vi "Motor_Plus_Impedance_controller_thursday.vi"() -> ()   [LabVIEW 2016]
uses:
  <vilib>/Platform/TimedLoop/XDataNode/timing_clust.ctl
  <vilib>/Platform/TimedLoop/XDataNode/nitl_modes.ctl
  <vilib>/Platform/TimedLoop/XDataNode/wakeup.ctl
  <vilib>/Platform/TimedLoop/XDataNode/loadnilvce.vi
  <vilib>/Motion/Express/_s/nimc.ax.power.power.axis.vi
  <vilib>/Motion/Express/_s/nimc.fb.read.readExecutionData.axis.vi
  <vilib>/Motion/Express/_s/nimc.fb.straightLineMove.startStraightLineMove.axis.modeVelocity.0.vi
  <vilib>/Motion/Express/_s/nimc.fb.stopMove.stop.axis.modeDecelerate.vi
  <vilib>/Motion/Express/_s/nimc.fb.resetPosition.resetPosition.axis.vi
  <vilib>/Motion/Express/_s/nimc.ex.power.power.axis.vi
  <vilib>/platform/TimedLoop/XDataNode/XDataNode.xnode
  <vilib>/Motion/BlockNode/FB.NIMotion.xnode
  <vilib>/Platform/TimedLoop/XDataNode/XDNodeRunTimeDep.lvlib
panel:
  in  "Exo Force 2":dbl=0.25 format="%#_13g"
  in  "Speed 2":dbl=0.25 format="%#_13g"
  in  "Position 2":dbl=0.25 format="%#_13g"
  in  "Exo Force":dbl=0.25 format="%#_13g"
  out "Adjusted Motor Velocity":dbl format="%.3f"
  out "Adjusted Velocity":dbl(knob) scale=0.0..3.0
  in  "Reset Position":bool
  in  "Position":dbl=0.25 format="%#_13g"
  in  "Speed":dbl=0.25 format="%#_13g"
  out "Torque":dbl(knob) scale=-5.0..5.0
  out "Position":dbl(knob) scale=0.0..1.0
  out "Velocity":dbl(knob) scale=0.0..5.0
  out "Load Cell":dbl(knob) scale=0.0..10.0
  in  "Move to Position?":bool
  out "Load cell, V":dbl format="%.3f"
  out "motor torque, Nm":dbl format="%.3f"
  out "motor velocity, rev/s":dbl format="%.3f"
  out "motor position, rev":dbl format="%.3f"
  in  "STOP VI":bool
  in  "Enable Axis \nControl":bool
  in  "Enable Motor \nDrive":bool
  in  "EMERGENCY MOTOR STOP":bool
  # "Raw Data from System"
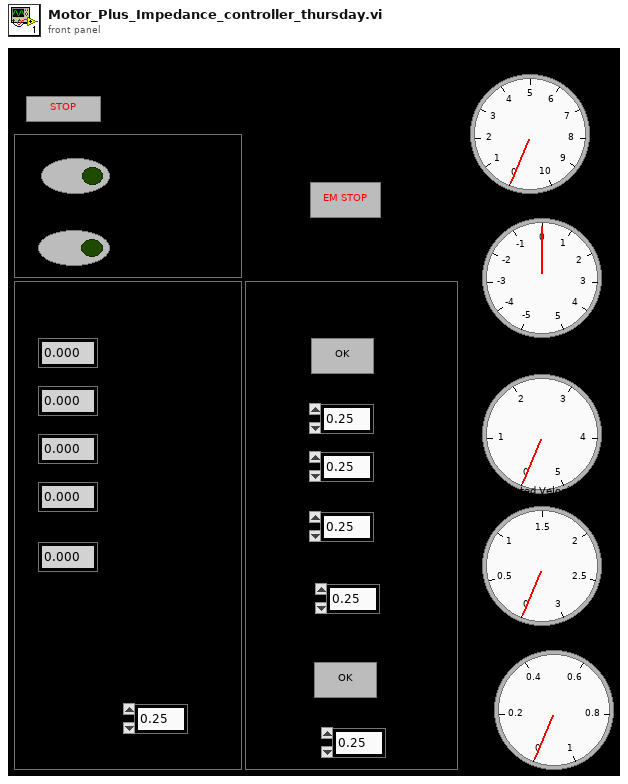
[diagram p1: front panel]
types:
  T1 = typedef "XDNodeRunTimeDep.lvlib/timing_clust.ctl" = cluster{"Expected End [f-1]":u64, "Actual End [f-1]":u64, "Finished Late? [f-1]":bool, "Expected End [i-1]":u64, "Actual End [i-1]":u64, "Finished Late? [i-1]":bool, "Expected Start [i]":u64, "Actual Start [i]":u64, "Expected Start [f]":u64, "Actual Start [f]":u64, "Source Name":string, "Structure Name":string, "Period":i64, "Deadline":i64, "Offset":i64, "Start":i64, "Priority":i32, "Timeout":i32, "Mode":T2, "Wakeup Reason":T3, "Error":errorcluster, "Source Type":string, "Secondary Source Type":string, "Global End Time":u64, "Global Start Time":u64, "Frame Duration":u64, "Iteration Duration":u64, "Assigned CPU":i32, "I/O Scan Engine Mode":u32}
  T2 = typedef "XDNodeRunTimeDep.lvlib/nitl_modes.ctl" = enum32{"No Change", "Process missed periods, maintain original phase", "Discard missed periods, maintain original phase", "Process missed periods, ignore original phase", "Discard missed periods, ignore original phase"}
  T3 = typedef "XDNodeRunTimeDep.lvlib/wakeup.ctl" = enum32{"Normal", "Aborted", "Asynchronous wakeup", "Timing source error", "Timed loop error", "Timeout"}
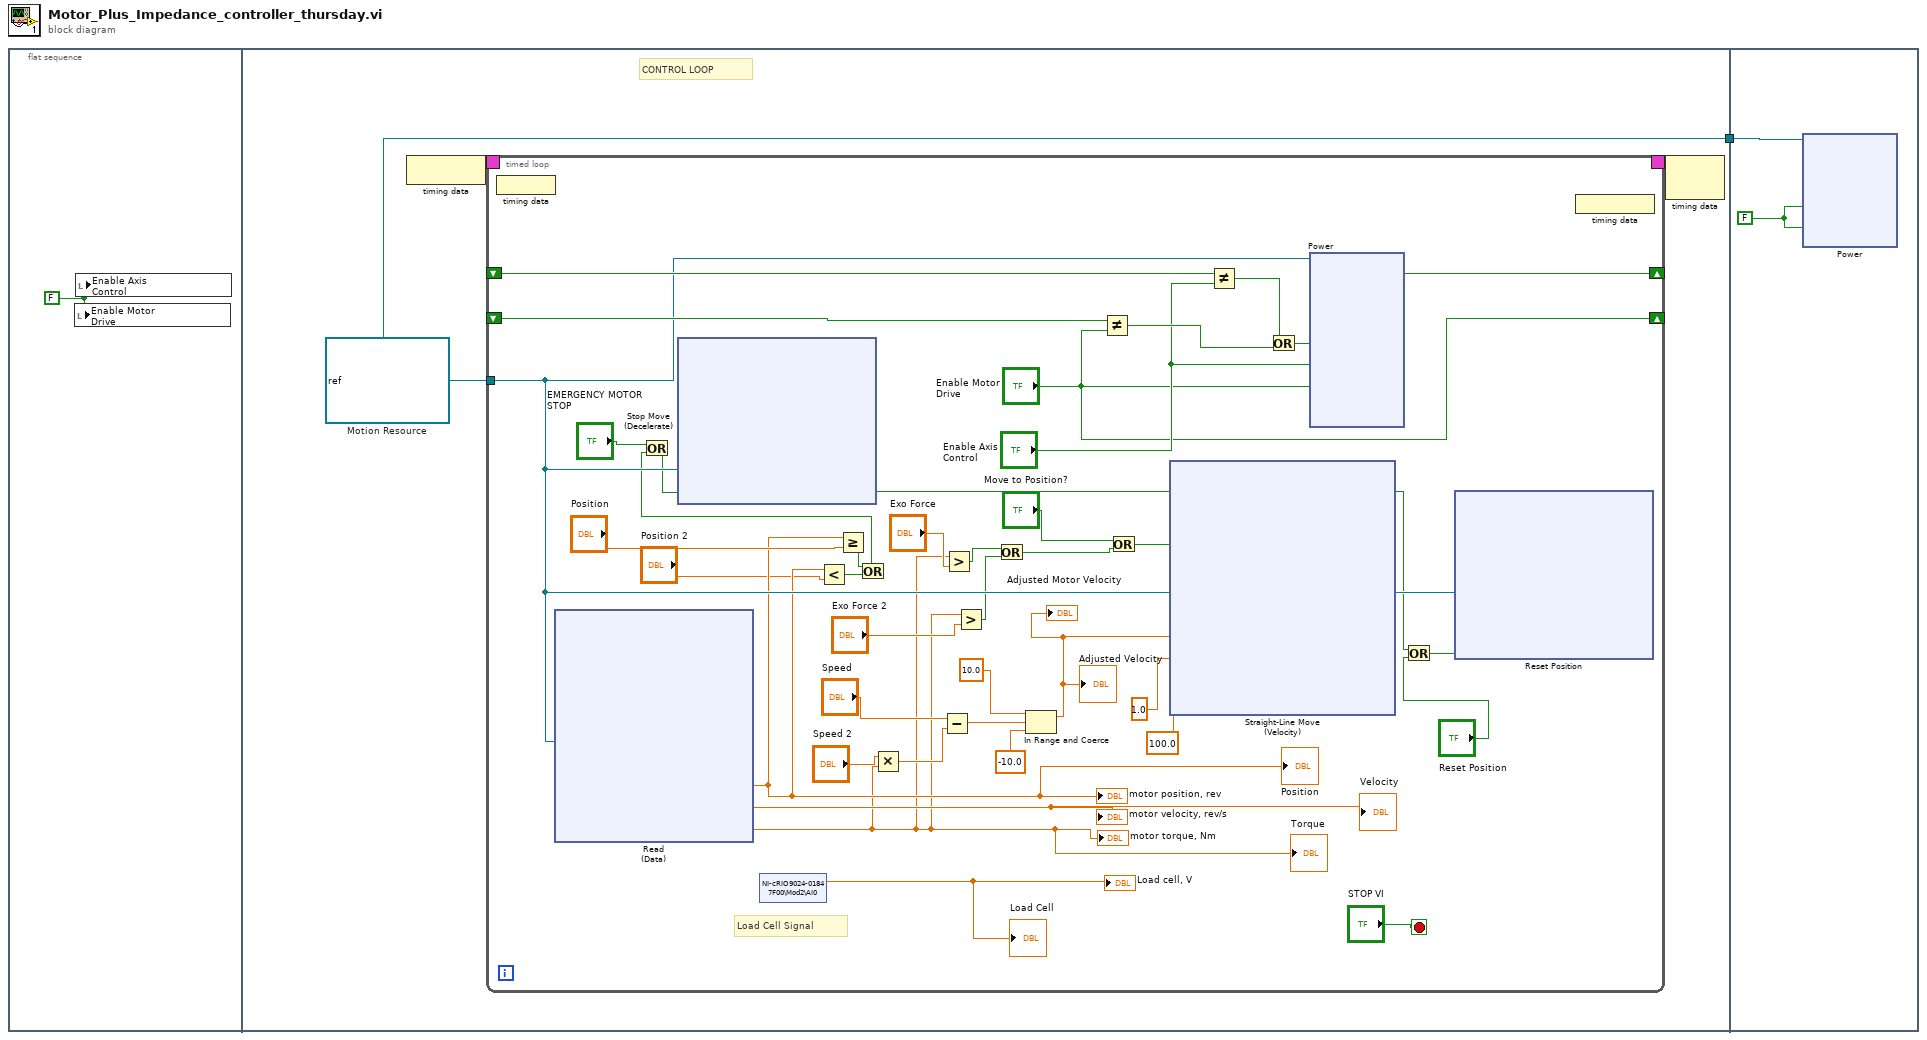
[diagram p0: block diagram]
diagram:
  n1 = flat-sequence {
    tunnel: [w5] -> w1
    tunnel: w1 -> [w123]
    frame #0 {
      w2 = FALSE
      n2 = local write "Enable Motor \nDrive"(w2) -> ()
      n3 = local write "Enable Axis \nControl"(w2) -> ()
    }
    frame #1 {
      w5 = refnum<k21> "nism://NI-cRIO9024-01847F00/Axis 1"  # Motion Resource
      # "CONTROL LOOP"
      n4 = node-c288() -> (w4:T1)
      n5 = timed-loop {
        tunnel: w5 -> [w36]
        timing: w4 -> [_]
        timing-out: [_] -> w3
        shift-right: ["Enable Axis \nControl"] -> _
        shift-left: _ -> [w44]
        shift-right: ["Enable Motor \nDrive"] -> _
        shift-left: _ -> [w43]
        stop <- "STOP VI" stop-if-true
        # "Load Cell Signal"
        n6 = node-c288() -> ()  [unwired: 1 in]
        n7 = xnode "Read\n(Data)"("resource"=w36) -> ("position"=w17:dbl, "torque"=w9:dbl, "velocity"=→"motor velocity, rev/s" →"Velocity":dbl)  [unwired: 1 in, 3 out]
        "motor position, rev" <- w17
        "motor torque, Nm" <- w9
        "Position" <- w17
        "Torque" <- w9
        n8 = shared-variable "NI-cRIO9024-01847F00\\Mod2\\AI0"() -> (→"Load cell, V" →"Load Cell":dbl)  [unwired: 1 in, 1 out]
        n9 = Less?(x=w17, y="Position 2") -> (x < y?=w15:bool)
        n10 = Greater Or Equal?(x=w17, y="Position") -> (x >= y?=w14:bool)
        n11 = Or(x=w14, y=w15) -> (x .or. y?=w13:bool)
        n12 = Or(x="EMERGENCY MOTOR STOP", y=w13) -> (x .or. y?=w25:bool)
        n13 = xnode "Stop Move\n(Decelerate)"("resource"=w36, "execute"=w25) -> ("done"=w28:bool)  [unwired: 1 in, 2 out]
        n14 = Multiply(x="Speed 2", y=w9) -> (x*y=w12:dbl)
        n15 = Subtract(x="Speed", y=w12) -> (x-y=w22:dbl)
        n16 = Greater?(x=w9, y="Exo Force") -> (0:w7:bool)
        n17 = Greater?(x=w9, y="Exo Force 2") -> (0:w6:bool)
        n18 = Or(x=w7, y=w6) -> (x .or. y?=w8:bool)
        n19 = In Range and Coerce(upper limit=10.0, x=w22, lower limit=-10.0) -> (coerced(x)=w27:dbl)  [unwired: 1 out]
        "Adjusted Velocity" <- w27
        "Adjusted Motor Velocity" <- w27
        n20 = Not Equal?(x=w43, y="Enable Motor \nDrive") -> (x != y?=w41:bool)
        n21 = Or(x="Move to Position?", y=w8) -> (x .or. y?=w20:bool)
        n22 = xnode "Straight-Line Move\n(Velocity)"("resource"=w36, "execute"=w20, "velocity"=w27, "acceleration"=1.0, "deceleration"=100.0) -> ("resource out"=w32:refnum<k21>)  [unwired: 1 in, 2 out]
        n23 = Not Equal?(x=w44, y="Enable Axis \nControl") -> (x != y?=w42:bool)
        n24 = Or(x=w42, y=w41) -> (x .or. y?=w40:bool)
        n25 = xnode ("Power")("execute"=w40, "enable axis"="Enable Axis \nControl", "enable drive"="Enable Motor \nDrive", "resource"=w36) -> ()  [unwired: 1 in, 6 out]
        n26 = Or(x=w28, y="Reset Position") -> (x .or. y?=w31:bool)
        n27 = xnode "Reset Position"("resource"=w32, "execute"=w31) -> ()  [unwired: 2 in, 3 out]
        n28 = node-c288() -> ()  [unwired: 1 out]
      }
      n29 = node-c288(w3) -> ()  [unwired: 1 out]
    }
    frame #2 {
      w124 = FALSE
      n30 = xnode ("Power")("enable axis"=w124, "enable drive"=w124, "resource"=w123) -> ()  [unwired: 1 in, 2 out]
    }
  }
